vi "Begin.vi"(8 "error in":errorcluster) -> (0 "error out":errorcluster)   [LabVIEW 2014]
doc: "Called before other user functions, this VI is expected to open initial I/O refnums, load in file data, and do all program initialization. Notice that the <B>error out</B> terminal is simply used for data flow. Wiring it to other structures or subVIs ensures that this VI runs first."
uses:
  <vilib>/Rock Robotics/WPI/DriverStation/WPI_DriverStationRobotMode2.ctl
  <vilib>/Rock Robotics/WPI/Joystick/WPI_JoystickDeviceEnum.ctl
  <vilib>/Rock Robotics/SystemInterfaces/DIO/FPGA_DIOPWMChannel.ctl
  <vilib>/Rock Robotics/WPI/CAN/TalonSRX/WPI_CANTalonSRX_APIFeedbackSelect.ctl
  <vilib>/Rock Robotics/WPI/CAN/TalonSRX/WPI_CANTalonSRX_APIControlMode.ctl
  <vilib>/Rock Robotics/WPI/SafetyOutput/WPI_SafetyOutputConfigMenu.ctl
  Robot Global Data.vi
  <vilib>/Rock Robotics/WPI/MotorControl/WPI_MotorControlOpen Jaguar.vi
  <vilib>/Rock Robotics/WPI/MotorControl/WPI_MotorControlOpenCANTalonSRX.vi
  <vilib>/Rock Robotics/WPI/MotorControl/WPI_MotorControlOpen Talon.vi
panel:
  in  "Ramp Rate":dbl=48.0 format="%#_13g"
  in  "I Zone":dbl=10.0 format="%#_13g"
  in  "Arm F":dbl format="%#_13g"
  in  "Arm D":dbl=9000.0 format="%#_13g"
  in  "Arm I":dbl=0.05 format="%#_13g"
  in  "Arm P":dbl=12.5 format="%#_13g"
  in  "Right Motors Inverted":bool=TRUE
  in  "Rear Left Motor":u8=2
  in  "Rear Right Motor":u8=4
  in  "Front Right Motor":u8=3
  in  "Front Left Motor":u8=1
  in  "Left Motors Inverted":bool=TRUE
  in  "Reverse Feedback Sensor":bool
  in  "I":dbl
  in  "F":dbl=0.01
  in  "D":dbl
  in  "P":dbl=1.0
  in  "Reverse Feedback Sensor":bool
  # "PID Options For Arm"
  # "RobotDrive Layout"
  # "PID Options for the Robot Drive"
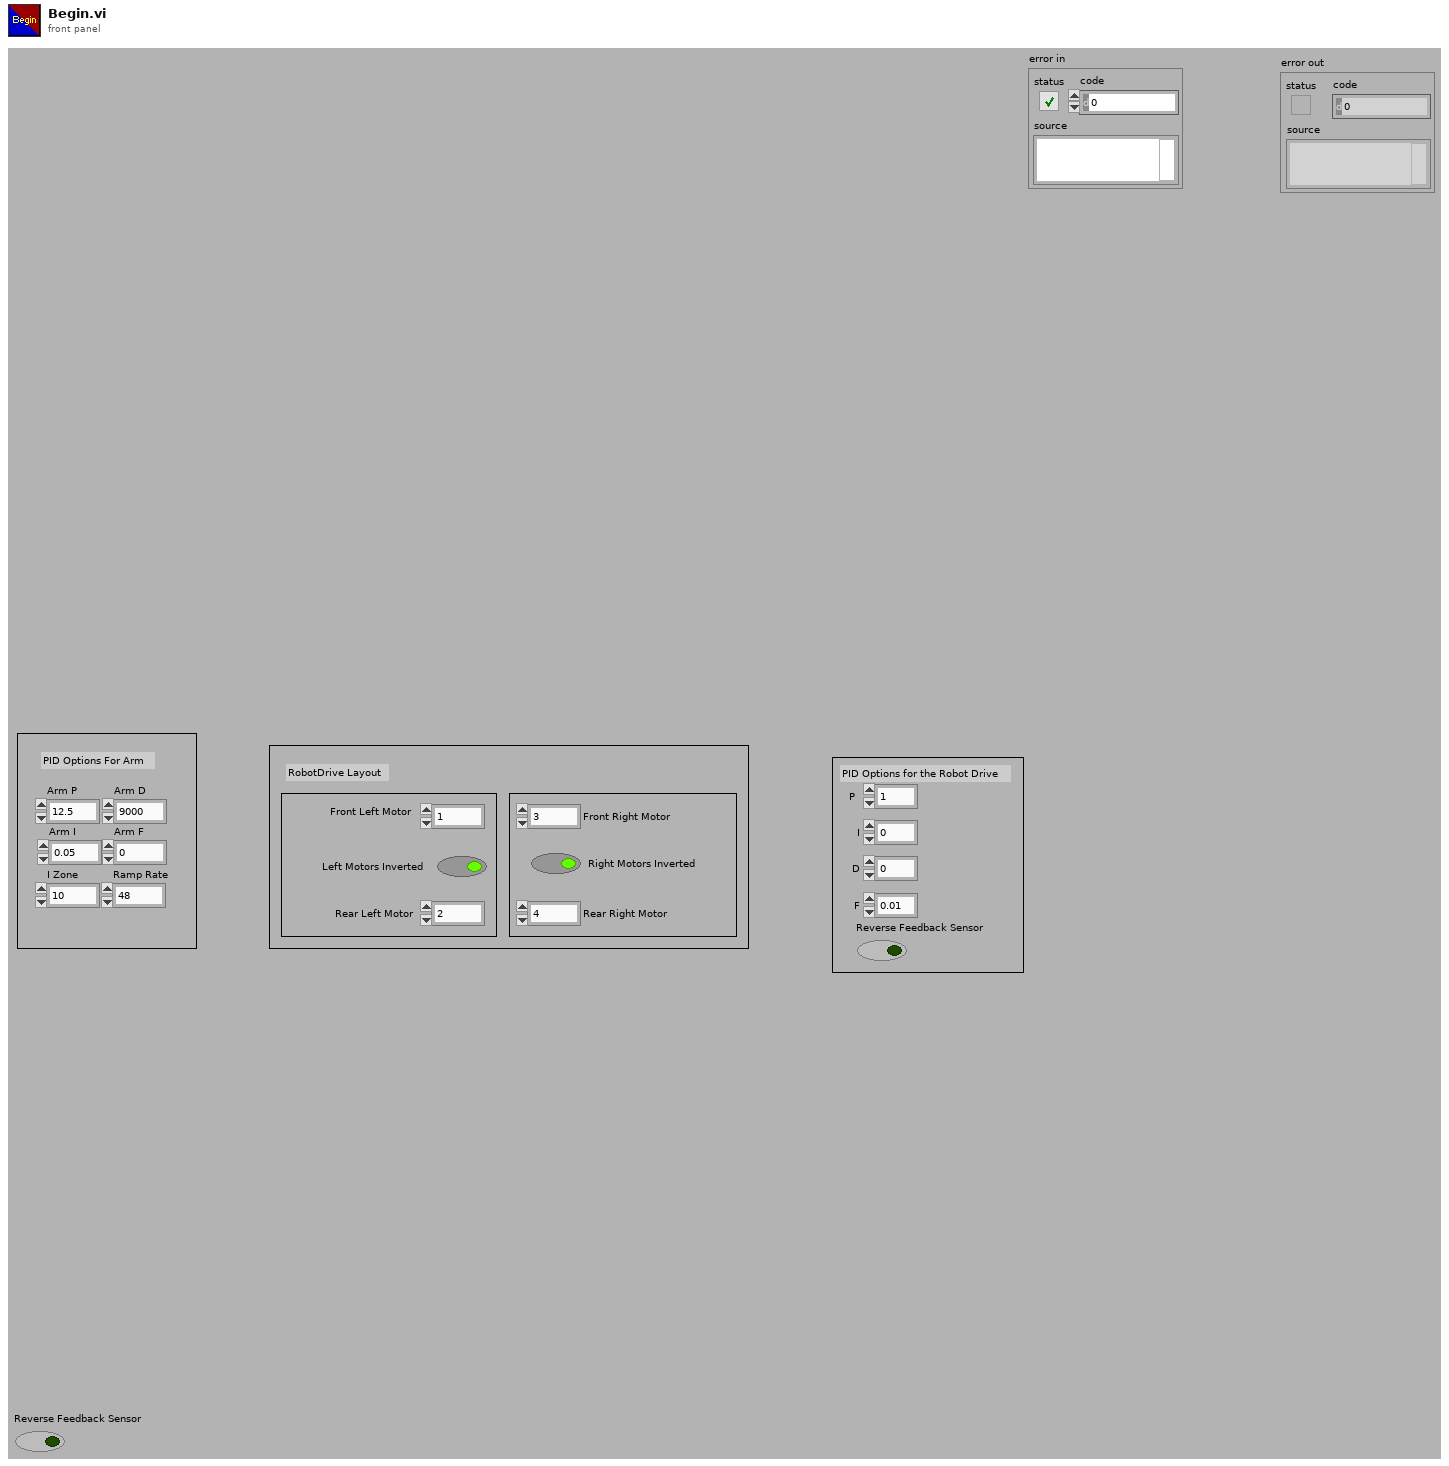
[diagram p1: front panel]
types:
  T1 = typedef "WPI_SafetyOutputConfigMenu.ctl" = enum16{"Enable", "Disable"}
  T2 = typedef "WPI_CANTalonSRX_APIControlMode.ctl" = enum8{"Percent VBus", "Speed", "Position", "Slave", "Unchanged / Invalid"}
  T3 = typedef "WPI_CANTalonSRX_APIFeedbackSelect.ctl" = enum16{"Digital Quadrature Encoder", "Analog Potentiometer", "Analog Encoder"}
  T4 = typedef "WPI_JoystickDeviceEnum.ctl" = enum16{"USB 0", "USB 1", "USB 2", "USB 3", "USB 4", "USB 5"}
  T5 = typedef "FPGA_DIOPWMChannel.ctl" = enum8{"PWM 0", "PWM 1", "PWM 2", "PWM 3", "PWM 4", "PWM 5", "PWM 6", "PWM 7", "PWM 8", "PWM 9", "PWM MXP 0", "PWM MXP 1", "PWM MXP 2", "PWM MXP 3", "PWM MXP 4", "PWM MXP 5", "PWM MXP 6", "PWM MXP 7", "PWM MXP 8", "PWM MXP 9", "Invalid"}
  T6 = typedef "WPI_DriverStationRobotMode2.ctl" = enum16{"Autonomous Disabled", "Autonomous Enabled", "Teleop Disabled", "Teleop Enabled", "Disconnected", "Finish", "Test Disabled", "Test Enabled", "Emergency Stopped"}
  T7 = typedef "WPI_MotorControlDeviceRef.ctl" = cluster{"DeviceStatus":errorcluster, "Type":T8, "PWM":cluster{"Controller":T9, "PWM Channel":T5, "DeadBand":T10}, "CAN":cluster{"Device Number":u8, "Control Mode":T11, "Semaphore":T12, "Max Vout":dbl, "TalonSRX Control Mode":T2}, "Invert":bool, "TransformRef":T13, "InvTransformRef":T13}
  T8 = typedef "WPI_MotorControlType.ctl" = enum16{"PWM", "CAN", "CANTalonSRX"}
  T9 = typedef "FPGA_TypedefDigitalModule.ctl" = enum16{"Controller 1"}
  T10 = typedef "WPI_PWMDeadband.ctl" = cluster{"Name":string, "maxPositivePwm":i32, "minPositivePwm":i32, "centerPwm":i32, "maxNegativePwm":i32, "minNegativePwm":i32, "angularRange":u16}
  T11 = typedef "WPI_CANJaguar_ControlMode.ctl" = enum8{"Percent VBus", "Current", "Speed", "Position", "Voltage"}
  T12 = typedef "Semaphore RefNum" = refnum<k1>
  T13 = typedef "WPI_PWMTransform_ConPane.ctl" = refnum<vi>
  T14 = typedef "WPI_RobotDriveDevRef.ctl" = cluster{"DevStatus":errorcluster, "Motors[]":T7[], "Square Inputs":bool, "Max Output":dbl}
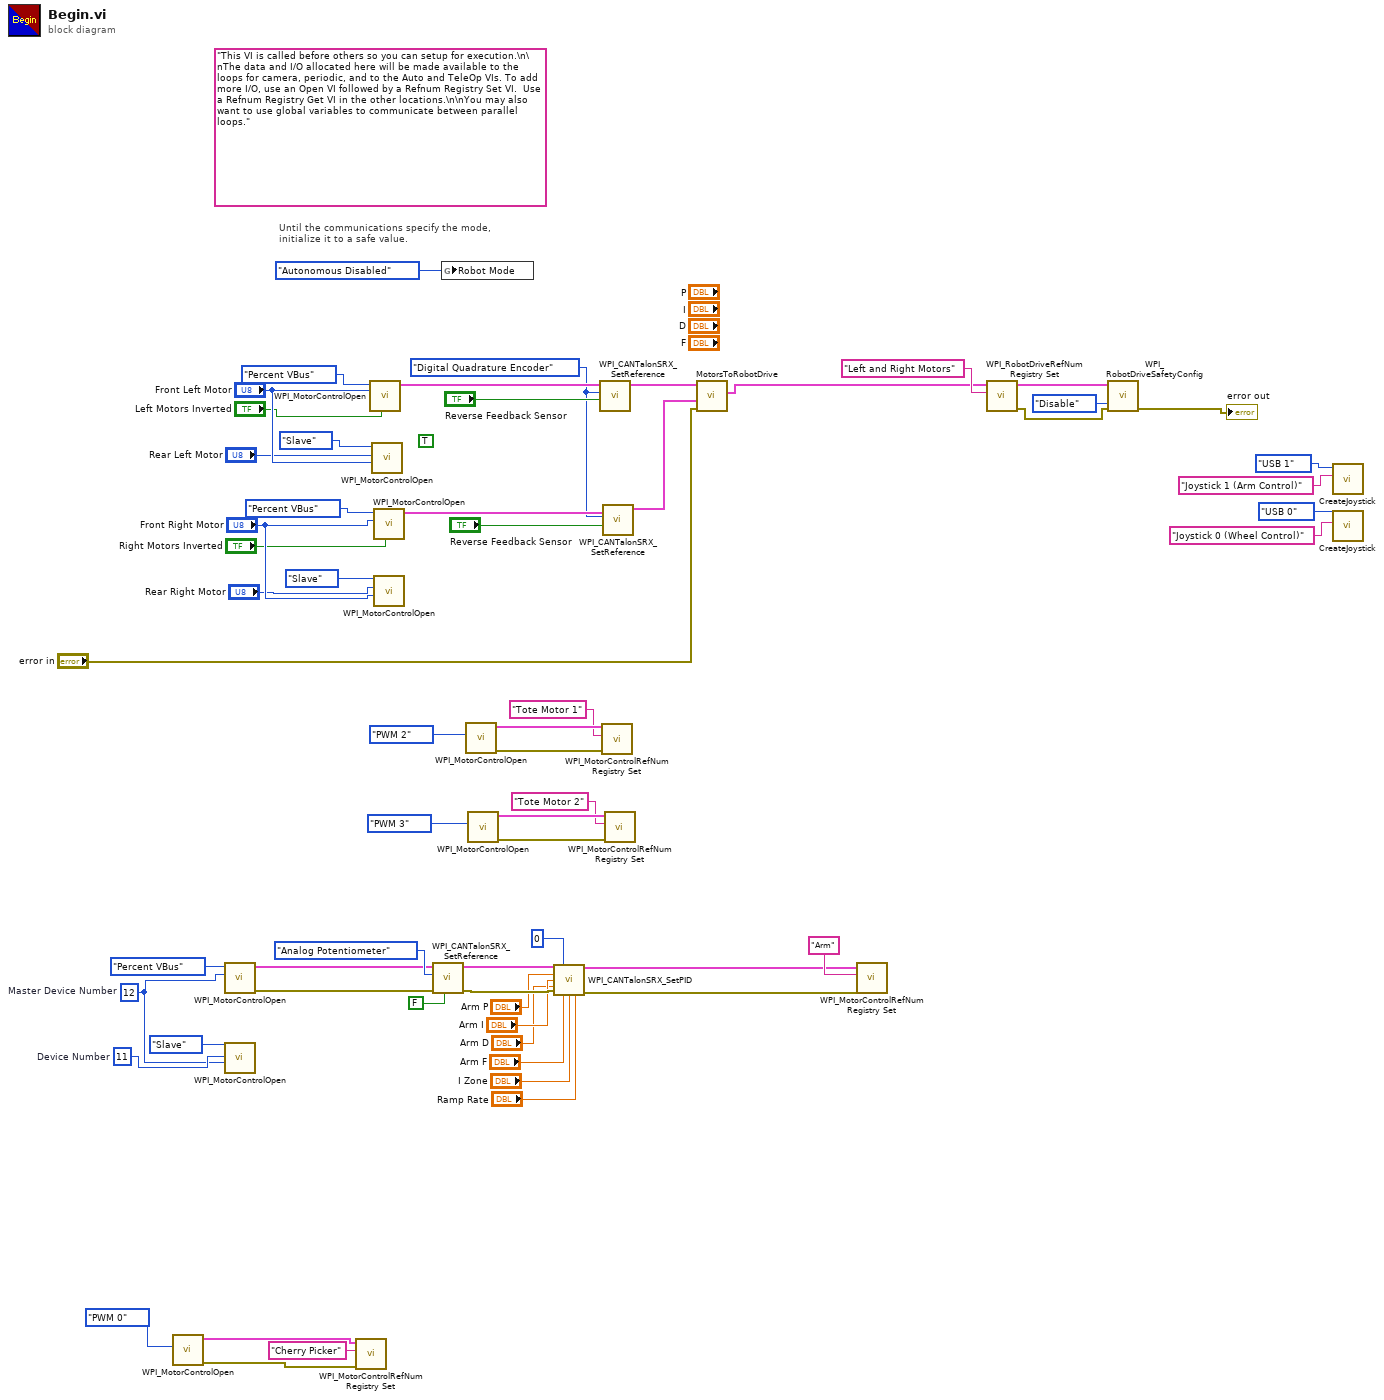
[diagram p0: block diagram]
diagram:
  (unwired) TRUE ("Left Motors Inverted")
  w7 = WPI_CANTalonSRX_APIFeedbackSelect."Digital Quadrature Encoder" ("Feedback Reference")
  w49 = u8 12  # Master Device Number
  w51 = u8 11  # Device Number
  (unwired) "This VI is called before others so you can setup for execution.\n\nThe data and I/O allocated here will be made available to the loops for camera, periodic, and to the Auto and TeleOp VIs. To add more I/O, use an Open VI followed by a Refnum Registry Set VI.  Use a Refnum Registry Get VI in the other locations.\n\nYou may also want to use global variables to communicate between parallel loops."
  # "Until the communications specify the mode,\ninitialize it to a safe value."
  n1 = call-poly <vilib>:"WPI_MotorControlOpen.vi"("PWM Channel"=FPGA_DIOPWMChannel."PWM 0") -> ("error out"=w59:errorcluster, "MotorControlDeviceRef"=w60:T7)  [unwired: 9 in]
  n2 = call-poly <vilib>:"WPI_MotorControlOpen.vi"("Device Number"=w49, "Control Mode"=WPI_CANTalonSRX_APIControlMode."Percent VBus") -> ("error out"=w50:errorcluster, "MotorControlDeviceRef"=w52:T7)  [unwired: 5 in, 3 out]
  n3 = call-poly <vilib>:"WPI_MotorControlOpen.vi"("Master Device Number"=w49, "Device Number"=w51, "Control Mode"=WPI_CANTalonSRX_APIControlMode."Slave") -> ()  [unwired: 4 in, 5 out]
  n4 = call <vilib>:"WPI_MotorControlRefNum Registry Set.vi"("error in (no error)"=w59, "refnum name"="Cherry Picker", "MotorControlDevRef"=w60) -> ()  [unwired: 7 in, 2 out]
  n5 = call-poly <vilib>:"WPI_MotorControlOpen.vi"("Invert"="Left Motors Inverted", "Device Number"="Front Left Motor", "Control Mode"=WPI_CANTalonSRX_APIControlMode."Percent VBus") -> ("MotorControlDeviceRef"=w26:T7)  [unwired: 4 in, 4 out]
  n6 = call-poly <vilib>:"WPI_MotorControlOpen.vi"("Master Device Number"="Front Left Motor", "Device Number"="Rear Left Motor", "Control Mode"=WPI_CANTalonSRX_APIControlMode."Slave") -> ()  [unwired: 4 in, 5 out]
  n7 = call-poly <vilib>:"WPI_MotorControlOpen.vi"("Invert"="Right Motors Inverted", "Device Number"="Front Right Motor", "Control Mode"=WPI_CANTalonSRX_APIControlMode."Percent VBus") -> ("MotorControlDeviceRef"=w22:T7)  [unwired: 4 in, 4 out]
  n8 = call-poly <vilib>:"WPI_MotorControlOpen.vi"("Master Device Number"="Front Right Motor", "Device Number"="Rear Right Motor", "Control Mode"=WPI_CANTalonSRX_APIControlMode."Slave") -> ()  [unwired: 4 in, 5 out]
  n9 = call <vilib>:"WPI_CANTalonSRX_SetReference.vi"("Reverse Closed-Loop Output"=FALSE, "error in (no error)"=w50, "Feedback Reference"=WPI_CANTalonSRX_APIFeedbackSelect."Analog Potentiometer", "CAN Talon SRX Ref"=w52) -> ("error out"=w48:errorcluster, "CAN Talon SRX Ref Out"=w45:T7)  [unwired: 6 in]
  n10 = global write "Robot Global Data.vi" "Robot Mode"(WPI_DriverStationRobotMode2."Autonomous Disabled" ("Robot Mode")) -> ()
  n11 = call-poly <vilib>:"WPI_MotorControlOpen.vi"("PWM Channel"=FPGA_DIOPWMChannel."PWM 2") -> ("error out"=w36:errorcluster, "MotorControlDeviceRef"=w37:T7)  [unwired: 9 in]
  n12 = call-poly <vilib>:"WPI_MotorControlOpen.vi"("PWM Channel"=FPGA_DIOPWMChannel."PWM 3") -> ("error out"=w32:errorcluster, "MotorControlDeviceRef"=w33:T7)  [unwired: 9 in]
  n13 = call <vilib>:"WPI_CANTalonSRX_SetPID.vi"("CAN Talon SRX Ref"=w45, "Parameter Slot"=u8 0, "P"="Arm P", "I"="Arm I", "D"="Arm D", "error in (no error)"=w48, "F"="Arm F", "I Zone"="I Zone", "Ramp Rate"="Ramp Rate") -> ("CAN Talon SRX Ref Out"=w46:T7, "error out"=w47:errorcluster)  [unwired: 5 in]
  n14 = call <vilib>:"WPI_CANTalonSRX_SetReference.vi"("Reverse Feedback Sensor"="Reverse Feedback Sensor", "Feedback Reference"=w7, "CAN Talon SRX Ref"=w26) -> ("CAN Talon SRX Ref Out"=w15:T7)  [unwired: 7 in, 1 out]
  n15 = call <vilib>:"WPI_MotorControlRefNum Registry Set.vi"("error in (no error)"=w36, "refnum name"="Tote Motor 1", "MotorControlDevRef"=w37) -> ()  [unwired: 7 in, 2 out]
  n16 = call <vilib>:"WPI_CANTalonSRX_SetReference.vi"("Reverse Feedback Sensor"="Reverse Feedback Sensor", "Feedback Reference"=w7, "CAN Talon SRX Ref"=w22) -> ("CAN Talon SRX Ref Out"=w12:T7)  [unwired: 7 in, 1 out]
  n17 = call <vilib>:"WPI_MotorControlRefNum Registry Set.vi"("error in (no error)"=w32, "refnum name"="Tote Motor 2", "MotorControlDevRef"=w33) -> ()  [unwired: 7 in, 2 out]
  n18 = call "MotorsToRobotDrive.vi"("Left Motor"=w15, "Right Motor"=w12, "error in"="error in") -> ("RobotDriveDevRef"=w1:T14)  [unwired: 6 in, 1 out]
  n19 = call <vilib>:"WPI_MotorControlRefNum Registry Set.vi"("error in (no error)"=w47, "refnum name"="Arm", "MotorControlDevRef"=w46) -> ()  [unwired: 7 in, 2 out]
  n20 = call <vilib>:"WPI_RobotDriveRefNum Registry Set.vi"("refnum name"="Left and Right Motors", "RobotDriveDevRef"=w1) -> ("error out"=w13:errorcluster, "RobotDriveDevRef"=w16:T14)  [unwired: 1 in, 7 out]
  n21 = call <vilib>:"WPI_RobotDriveSafetyConfig.vi"("error in (no error)"=w13, "mode"=WPI_SafetyOutputConfigMenu."Disable", "RobotDriveDevRef"=w16) -> ("error out"=→"error out":errorcluster)  [unwired: 7 in, 1 out]
  n22 = call "CreateJoystick.vi"("refnum name"="Joystick 1 (Arm Control)", "JoystickDevice"=WPI_JoystickDeviceEnum."USB 1") -> ()  [unwired: 6 in, 2 out]
  n23 = call "CreateJoystick.vi"("refnum name"="Joystick 0 (Wheel Control)", "JoystickDevice"=WPI_JoystickDeviceEnum."USB 0") -> ()  [unwired: 6 in, 2 out]
